vi "Set Setpoint Value.vi"(7 "Unit Address (1)":u8=1, 8 "error in (no error)":errorcluster, 9 "Setpoint Value (0)":i16, 10 "Selected Setpoint (0: Setpoint 1)":u8(ring) items=["Setpoint 1", "Setpoint 2", "Alternate Setpoint", "Target Setpoint"], 11 "VISA resource name":refnum<visa-resource-name>) -> (0 "error out":errorcluster, 3 "VISA resource name out":refnum<visa-resource-name>)   [LabVIEW 2014, in "Eurotherm 35xx Series.lvlib"]
doc: "This VI sets setpoint value."
uses:
  <instrlib>/Eurotherm 35xx Series/Eurotherm 35xx Series.lvlib
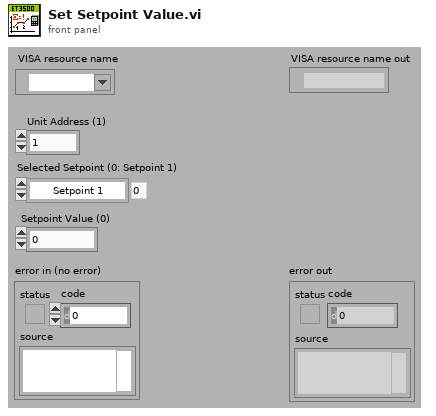
[diagram p1: front panel]
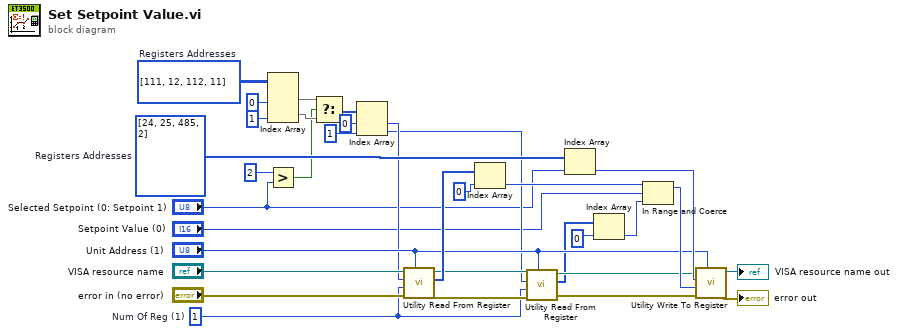
[diagram p0: block diagram]
diagram:
  w23 = u16[][] [[111, 12], [112, 11]]  # Registers Addresses
  w8 = u16 1  # Num Of Reg (1)
  w26 = u16[] [24, 25, 485, 2]  # Registers Addresses
  n1 = Index Array(array=w23, index (col) #1=0 ("disabled index (col)"), index (col) #2=1 ("index (col)")) -> (element #1=w20:u16[], element #2=w19:u16[])  [unwired: 2 in]
  n2 = Greater?(x=u8 2, y="Selected Setpoint (0: Setpoint 1)") -> (0:w1:bool)
  n3 = Select(t=w20, s=w1, f=w19) -> (s? t:f=w13:u16[])
  n4 = Index Array(array=w13, index #1=0 ("index"), index #2=1 ("index")) -> (element #1=w10:u16, element #2=w9:u16)
  n5 = call <instrlib>:"Utility Read From Register.vi"("Unit Address (1)"="Unit Address (1)", "error in (no error)"="error in (no error)", "Num Of Reg (1)"=w8, "Register Address (0)"=w10, "VISA resource name"="VISA resource name") -> ("error out"=w15:errorcluster, "Data"=w31:i16[], "VISA resource name out"=w18:refnum<visa-resource-name>)  [unwired: 4 in]
  n6 = Index Array(array=w31, index=0) -> (element=w29:i16)
  n7 = call <instrlib>:"Utility Read From Register.vi"("Unit Address (1)"="Unit Address (1)", "error in (no error)"=w15, "Num Of Reg (1)"=w8, "Register Address (0)"=w9, "VISA resource name"=w18) -> ("error out"=w16:errorcluster, "Data"=w6:i16[], "VISA resource name out"=w17:refnum<visa-resource-name>)  [unwired: 4 in]
  n8 = Index Array(array=w26, index="Selected Setpoint (0: Setpoint 1)") -> (element=w25:u16)
  n9 = Index Array(array=w6, index=0) -> (element=w5:i16)
  n10 = In Range and Coerce(upper limit=w29, x="Setpoint Value (0)", lower limit=w5) -> (coerced(x)=w24:i16)  [unwired: 1 out]
  n11 = call <instrlib>:"Utility Write To Register.vi"("Unit Address (1)"="Unit Address (1)", "error in (no error)"=w16, "Data (0)"=w24, "Register Address (0)"=w25, "VISA resource name"=w17) -> ("error out"=→"error out":errorcluster, "VISA resource name out"=→"VISA resource name out":refnum<visa-resource-name>)  [unwired: 5 in]
